vi "Get Meta Data.vi"(8 "error in":errorcluster, 11 "VISA Interface in":refnum<class "VISA Interface.lvclass">) -> (0 "error out":errorcluster, 2 "Get Meta Data":T1, 3 "VISA Interface out":refnum<class "VISA Interface.lvclass">)   [LabVIEW 2020, in "Plugin Instrument Driver.lvlib" / "VISA Interface.lvclass"]
doc: "This is a placeholder API to get Meta data details"
uses:
  VISA Interface.lvclass
  builds/Libraries/Shared GUI Library.lvlibp/Shared GUI Library/Device Meta Data Cluster/Get Meta Data.ctl
  builds/Libraries/Shared GUI Library.lvlibp
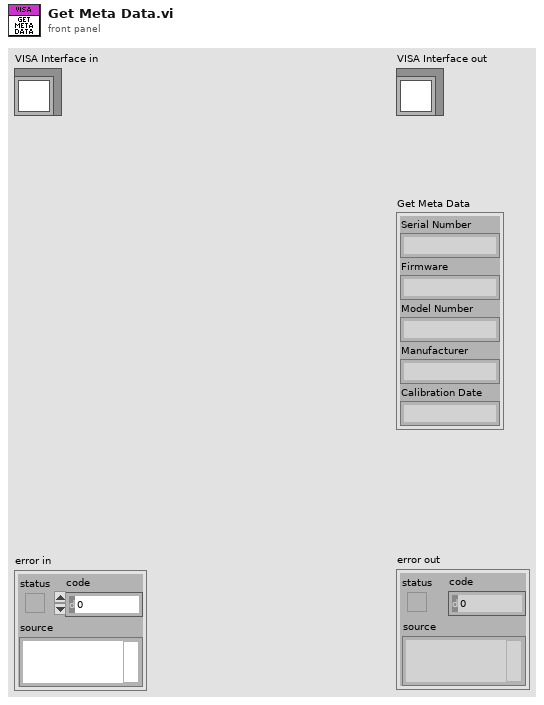
[diagram p1: front panel]
types:
  T1 = typedef "Shared GUI Library.lvlibp/Get Meta Data.ctl" = cluster{"Serial Number":string, "Firmware":string, "Model Number":string, "Manufacturer":string, "Calibration Date":string}
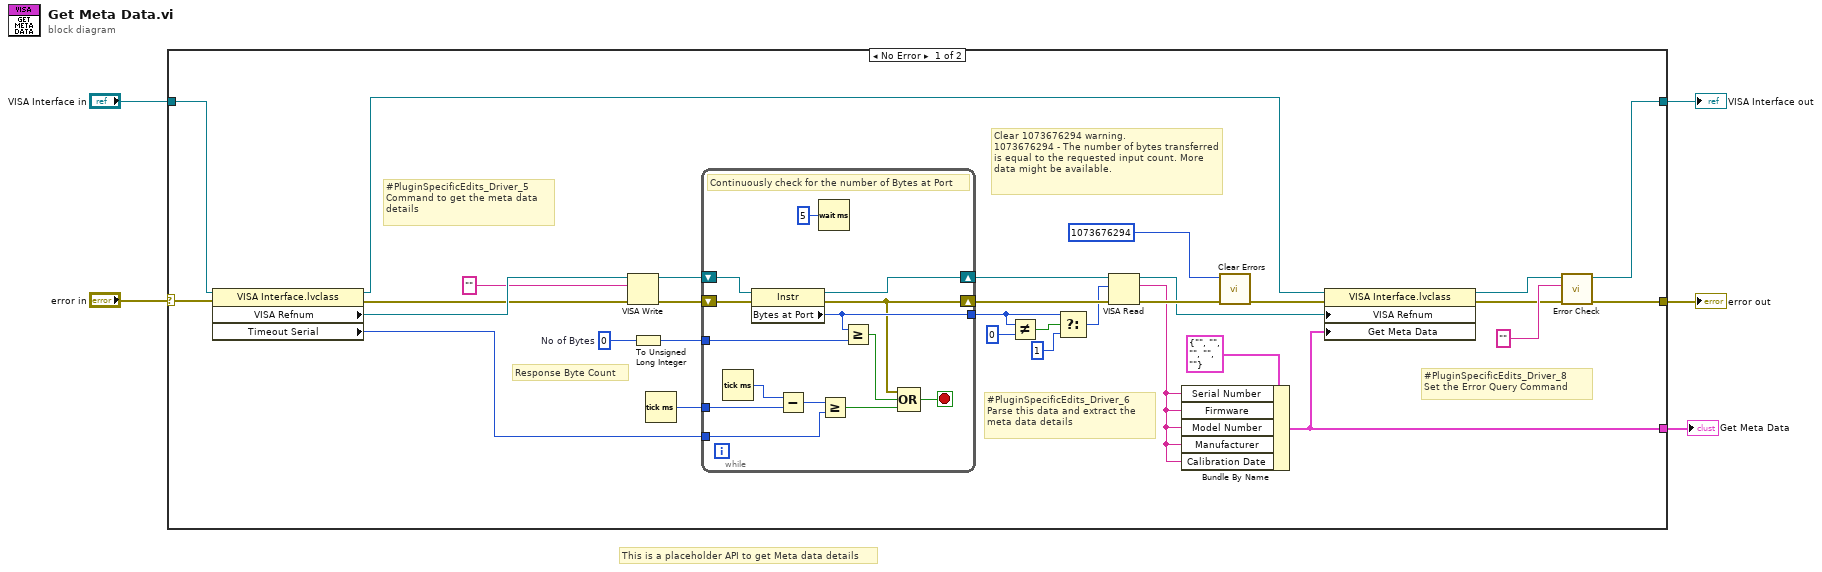
[diagram p0: block diagram]
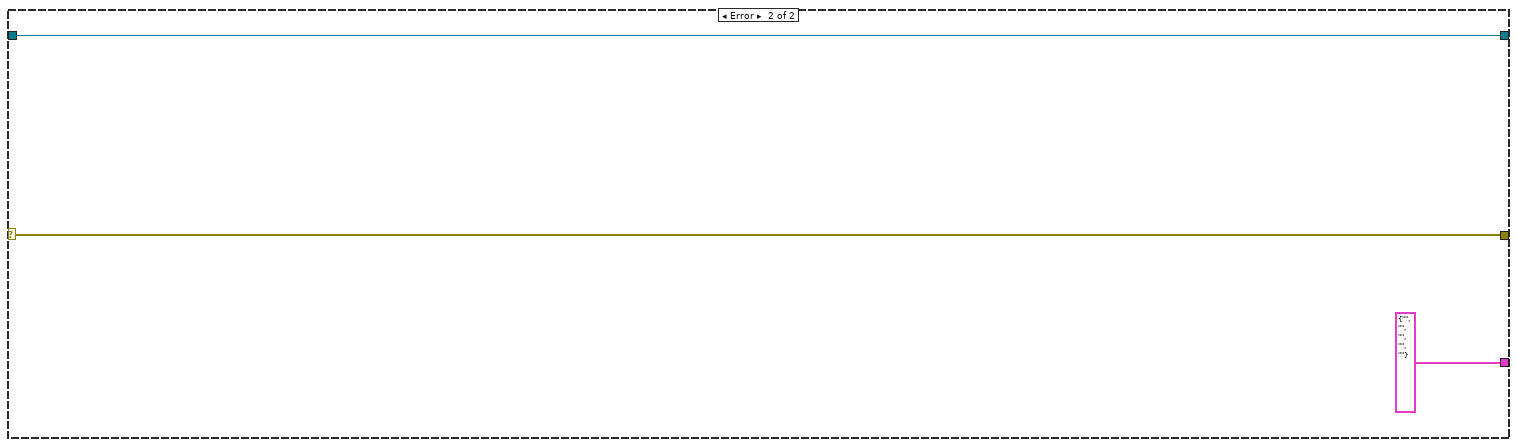
[diagram p2: hidden frame]
diagram:
  # "This is a placeholder API to get Meta data details"
  n1 = case shown="No Error" "error in" {
    selector: "error in" -> [w20 w52]
    tunnel: [w14 w53] -> w3
    tunnel: "VISA Interface in" -> [w21 w53]
    tunnel: [w13 w52] -> w2
    tunnel: [w6 T1 {"Serial Number"="", "Firmware"="", "Model Number"="", "Manufacturer"="", "Calibration Date"=""} ("Get Meta Data")] -> w1
    frame No Error {
      w25 = u32 0  # No of Bytes
      # "#PluginSpecificEdits_Driver_8 \nSet the Error Query Command"
      # "#PluginSpecificEdits_Driver_6 \nParse this data and extract the\nmeta data details"
      # "#PluginSpecificEdits_Driver_5 \nCommand to get the meta data\ndetails"
      # "Clear 1073676294 warning.\n1073676294 - The number of bytes transferred is equal to the requested input count. More data might be available."
      # "Response Byte Count"
      n2 = property class="VISA Interface.lvclass"(reference=w21, error in=w20) -> (reference out=w11:refnum<class "VISA Interface.lvclass">, error out=w18:errorcluster, "VISA Refnum"=w19:refnum<visa-resource-name>, "Timeout Serial"=w24:u32)
      n3 = VISA Write(VISA resource name=w19, write buffer="", error in (no error)=w18) -> (VISA resource name out=w34:refnum<visa-resource-name>, error out=w36:errorcluster)  [unwired: 1 out]
      n4 = To Unsigned Long Integer(number=w25) -> (unsigned 32bit integer=w31:u32)
      n5 = Tick Count (ms)() -> (millisecond timer value=w32:u32)
      n6 = while {
        tunnel: [w47] -> w26
        shift-right: [w42] -> w35
        shift-left: w36 -> [w50]
        shift-right: [w48] -> w33
        shift-left: w34 -> [w49]
        tunnel: w32 -> [w44]
        tunnel: w31 -> [w38]
        tunnel: w24 -> [w37]
        stop <- w39 stop-if-true
        # "Continuously check for the number of Bytes at Port"
        n7 = Tick Count (ms)() -> (millisecond timer value=w45:u32)
        n8 = property class="Instr"(reference=w49, error in=w50) -> (reference out=w48:refnum<visa-resource-name>, error out=w42:errorcluster, "Bytes at Port"=w47:u32)
        n9 = Subtract(x=w45, y=w44) -> (x-y=w43:u32)
        n10 = Wait (ms)(milliseconds to wait=u32 5) -> ()  [unwired: 1 out]
        n11 = Greater Or Equal?(x=w43, y=w37) -> (x >= y?=w40:bool)
        n12 = Greater Or Equal?(x=w47, y=w38) -> (x >= y?=w41:bool)
        n13 = Compound Arithmetic op=OR(w42, w41, w40) -> (w39:bool)
      }
      n14 = Not Equal?(x=w26, y=u32 0) -> (x != y?=w29:bool)
      n15 = Select(t=w26, s=w29, f=u32 1 ("t")) -> (s? t:f=w28:u32)
      n16 = VISA Read(VISA resource name=w33, byte count=w28, error in (no error)=w35) -> (VISA resource name out=w9:refnum<visa-resource-name>, read buffer=w15:string, error out=w22:errorcluster)  [unwired: 1 out]
      n17 = Bundle By Name(cluster=T1 {"Serial Number"="", "Firmware"="", "Model Number"="", "Manufacturer"="", "Calibration Date"=""} ("Get Meta Data"), "Serial Number"=w15, "Firmware"=w15, "Model Number"=w15, "Manufacturer"=w15, "Calibration Date"=w15) -> (w6:T1)
      n18 = call <vilib>:"Clear Errors.vi"("error in (no error)"=w22, "specific error code to clear (0: all)"=1073676294) -> ("error out"=w8:errorcluster)  [unwired: 4 in, 1 out]
      n19 = property class="VISA Interface.lvclass"(reference=w11, error in=w8, "VISA Refnum"=w9, "Get Meta Data"=w6) -> (reference out=w10:refnum<class "VISA Interface.lvclass">, error out=w7:errorcluster)
      n20 = call "Error Check.vi"("error in"=w7, "Error Query Command"="", "VISA Interface in"=w10) -> ("error out"=w13:errorcluster, "VISA Interface out"=w14:refnum<class "VISA Interface.lvclass">)  [unwired: 7 in]
    }
    frame Error {
    }
  }
  "error out" <- w2
  "VISA Interface out" <- w3
  "Get Meta Data" <- w1
